vi "Multiclamp Set Holding Potential.vi"(7 "On":bool, 8 "error in (no error)":errorcluster, 9 "Voltage":dbl, 10 "pnError":i32, 11 "hMCCmsg":i32) -> (0 "error out":errorcluster, 2 "pnError out":i32, 3 "hMCCmsg OUT":i32)   [LabVIEW 2012, in "MultiClamp 700B Controls.lvlib"]
uses:
  MultiClamp 700B Controls.lvlib
  AxMultiClampMsg/AxMultiClampMsg.lvlib
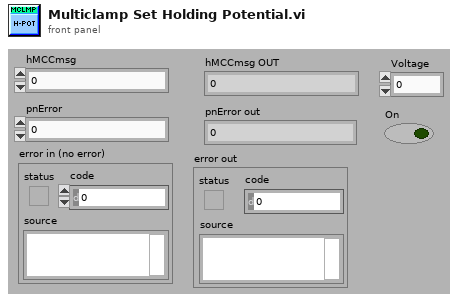
[diagram p1: front panel]
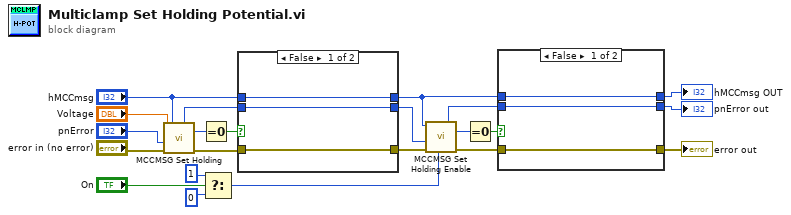
[diagram p0: block diagram]
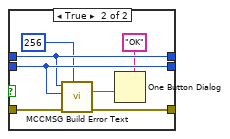
[diagram p2: hidden frame]
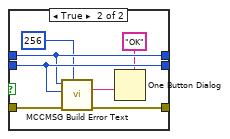
[diagram p3: hidden frame]
diagram:
  n1 = call "MCCMSG Set Holding.vi"("error in (no error)"="error in (no error)", "pnError"="pnError", "dHolding"="Voltage", "hMCCmsg"="hMCCmsg") -> ("error out"=w21:errorcluster, "pnError out"=w19:i32, "function return"=w20:i32)  [unwired: 5 in]
  n2 = Equal To 0?(x=w20) -> (x = 0?=w22:bool)
  n3 = Select(t=1, s="On", f=0 ("bEnable")) -> (s? t:f=w4:i32)
  n4 = case shown="False" w22 {
    tunnel: w19 -> [w25 w31]
    tunnel: w21 -> [w23 w32]
    tunnel: "hMCCmsg" -> [w24 w30]
    tunnel: [w25 w31] -> w12
    tunnel: [w24 w30] -> w13
    tunnel: [w23 w26] -> w14
    frame False {
    }
    frame True {
      n5 = call "MCCMSG Build Error Text.vi"("uMaxLen"=u32 256, "error in (no error)"=w32, "nErrorNum"=w31, "hMCCmsg"=w30) -> ("error out"=w26:errorcluster, "sTxtBuf out"=w29:string)  [unwired: 5 in, 1 out]
      n6 = One Button Dialog(message=w29, button name ("OK")="OK") -> ()  [unwired: 1 out]
    }
  }
  n7 = call "MCCMSG Set Holding Enable.vi"("error in (no error)"=w14, "pnError"=w12, "bEnable"=w4, "hMCCmsg"=w13) -> ("error out"=w16:errorcluster, "pnError out"=w15:i32, "function return"=w17:i32)  [unwired: 5 in]
  n8 = Equal To 0?(x=w17) -> (x = 0?=w18:bool)
  n9 = case shown="False" w18 {
    tunnel: w15 -> [w35 w41]
    tunnel: w16 -> [w33 w42]
    tunnel: w13 -> [w34 w40]
    tunnel: [w35 w41] -> w2
    tunnel: [w34 w40] -> w3
    tunnel: [w33 w36] -> w1
    frame False {
    }
    frame True {
      n10 = call "MCCMSG Build Error Text.vi"("uMaxLen"=u32 256, "error in (no error)"=w42, "nErrorNum"=w41, "hMCCmsg"=w40) -> ("error out"=w36:errorcluster, "sTxtBuf out"=w39:string)  [unwired: 5 in, 1 out]
      n11 = One Button Dialog(message=w39, button name ("OK")="OK") -> ()  [unwired: 1 out]
    }
  }
  "hMCCmsg OUT" <- w3
  "pnError out" <- w2
  "error out" <- w1
